vi "readyButton.vi"() -> (2 "Ready? 2":bool)   [LabVIEW 2017]
panel:
  in  "Ready?":bool
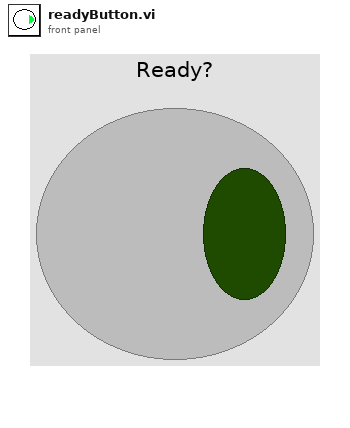
[diagram p1: front panel]
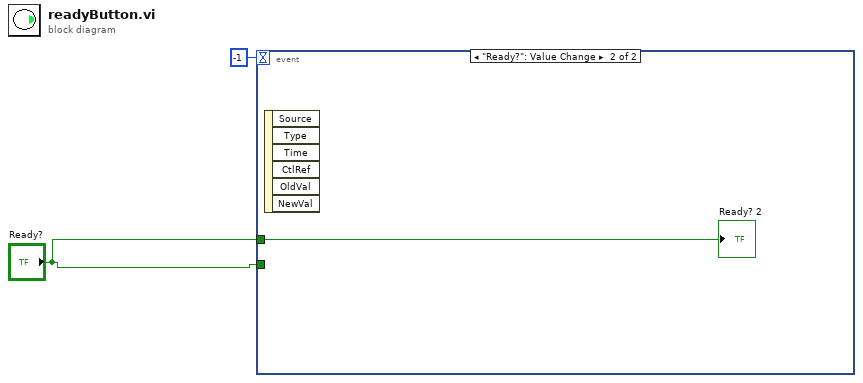
[diagram p0: block diagram]
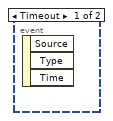
[diagram p2: hidden frame]
diagram:
  n1 = event shown="[1] \"Ready?\": Value Change" {
    selector: _ -> [_ _]
    dyn-events: _ -> [_ _]
    timeout: -1 -> [_ _]
    tunnel: "Ready?" -> [_ _]
    tunnel: "Ready?" -> [_ w3]
    event Timeout {
      n2 = event-data() -> ()  [unwired: 1 in, 3 out]
    }
    event "Ready?": Value Change {
      n3 = event-data() -> ()  [unwired: 1 in, 6 out]
      "Ready? 2" <- w3
    }
  }
